vi "parse_channel_list.vi"(8 "error in (no error)":errorcluster, 11 "HSDIO in":refnum<class "HSDIO.lvclass">) -> (0 "error out":errorcluster, 3 "HSDIO out":refnum<class "HSDIO.lvclass">)   [LabVIEW 2013, in "HSDIO.lvclass"]
uses:
  HSDIO.lvclass
panel:
  out "# active channels":u8
  out "Idle State (Binary)":u32 format="%b"
  out "Active Channels (String)":string
  out "decimal array":u8[](array[numeric])
  out "boolean array":bool[](array[boolean])
  out "Active Channels (Binary)":u32 format="%b"
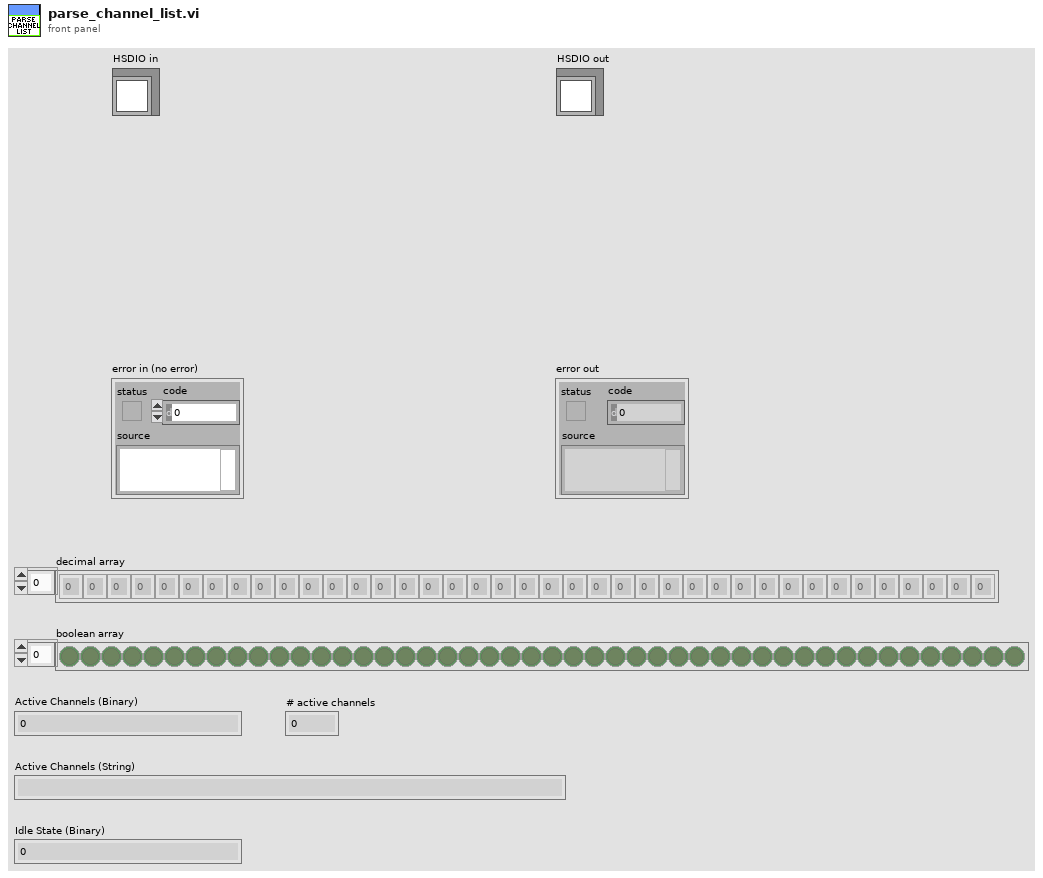
[diagram p1: front panel]
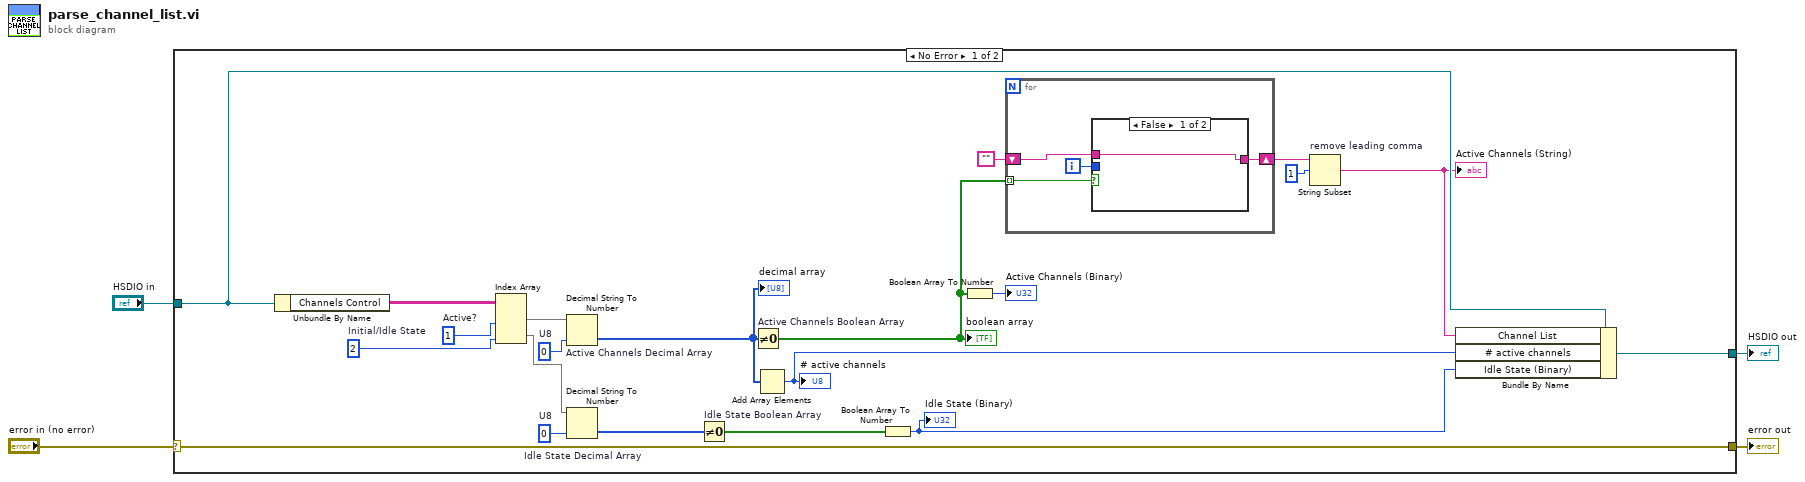
[diagram p0: block diagram]
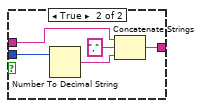
[diagram p2: hidden frame]
diagram:
  n1 = case shown="No Error" "error in (no error)" {
    selector: "error in (no error)" -> [w25 w37]
    tunnel: [w25 w37] -> w3
    tunnel: [w8 w36] -> w1
    tunnel: "HSDIO in" -> [w9 w36]
    frame No Error {
      w15 = 2  # Initial/Idle State
      w17 = u8 0  # U8
      w22 = 1  # Active?
      w23 = u8 0  # U8
      n2 = Unbundle By Name(w9) -> ("Channels Control"=w10:string[][])
      n3 = Index Array(array=w10, index (col) #1=w22, index (col) #2=w15) -> (element #1=w21:string[], element #2=w14:string[])  [unwired: 2 in]
      n4 = Decimal String To Number "Active Channels Decimal Array"(string=w21, default (0L)=w23) -> (number=w11:u8[])  [unwired: 1 in, 1 out]
      "decimal array" <- w11
      n5 = Decimal String To Number "Idle State Decimal Array"(string=w14, default (0L)=w17) -> (number=w16:u8[])  [unwired: 1 in, 1 out]
      n6 = Not Equal To 0? "Idle State Boolean Array"(x=w16) -> (x != 0?=w12:bool[])
      n7 = Not Equal To 0? "Active Channels Boolean Array"(x=w11) -> (x != 0?=w13:bool[])
      "boolean array" <- w13
      n8 = Add Array Elements(numeric array=w11) -> (sum=w7:u8)
      "# active channels" <- w7
      n9 = Boolean Array To Number(Boolean array=w12) -> (number=w6:u32)
      "Idle State (Binary)" <- w6
      n10 = Boolean Array To Number(Boolean array=w13) -> (number=→"Active Channels (Binary)":u32)
      n11 = for {
        tunnel: w13 -> [w26] mode=indexing
        shift-right: [w27] -> w19
        shift-left: "" -> [w29]
        i -> [w28]
        n12 = case shown="False" w26 {
          tunnel: w29 -> [w30 w35]
          tunnel: w28 -> [_ w34]
          tunnel: [w30 w33] -> w27
          frame False {
          }
          frame True {
            n13 = Number To Decimal String(number=w34) -> (decimal integer string=w32:string)  [unwired: 1 in]
            n14 = Concatenate Strings(w35, ",", w32) -> (w33:string)
          }
        }
      }
      n15 = String Subset "remove leading comma"(string=w19, offset (0)=1) -> (substring=w5:string)  [unwired: 1 in]
      "Active Channels (String)" <- w5
      n16 = Bundle By Name(cluster=w9, "Channel List"=w5, "# active channels"=w7, "Idle State (Binary)"=w6) -> (w8:refnum<class "HSDIO.lvclass">)
    }
    frame Error {
    }
  }
  "error out" <- w3
  "HSDIO out" <- w1
